vi "NIIE_LoadGraphics.vi"(4 "Templates User Event":refnum<user-event>, 6 "Glyphs User Event":refnum<user-event>, 8 "Error":errorcluster, 9 "Source":T1=enum."Icon Templates VI", 10 "Check Template?":bool, 11 "Graphic Root Folder":path) -> (0 "Error Out":errorcluster, 3 "Glyphs Out":T2[](array[typedef]), 5 "Match? Out":bool, 7 "Match Index Out":i32)   [LabVIEW 2021]
uses:
  MB CORE/TypeDefs/Cluster_Path&Icon.ctl
  vi.lib/LabVIEW Icon API/lv_icon/Controls/Pathes.ctl
  MB CORE/TypeDefs/Cluster_IconFilename.ctl
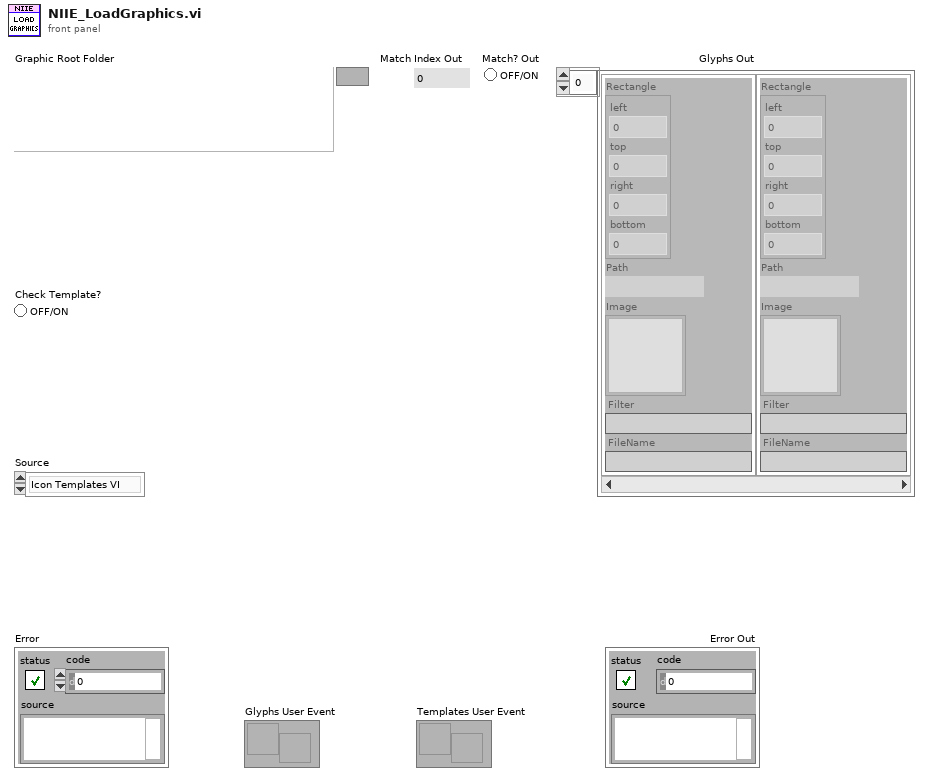
[diagram p1: front panel]
types:
  T1 = typedef "Pathes.ctl" = enum16{"Root Path", "Icon Templates", "Icon Templates VI", "Icon Templates Lib", "Glyphs"}
  T2 = typedef "Cluster_Path&Icon.ctl" = cluster{"Rectangle":cluster{"left":i16, "top":i16, "right":i16, "bottom":i16}, "Path":path, "Image":picture, "Filter":string, "FileName":string}
  T3 = typedef "Cluster_IconFilename.ctl" = cluster{"Name":string, "File Extension  ":string, "Filter":string, "Path":path}
  T4 = typedef "LabVIEW Icon Stored Information.ctl" = cluster{"Text Visible?":bool, "Text Opacity":u8, "Templ Visible?":bool, "Templ Opacity":u8, "Relative Path from 1 to 2":path, "Image":picture, "All User Layers":refnum<class "Layer.lvclass">[], "Body Text":T5}
  T5 = typedef "Cluster_BodyText.ctl" = cluster{"Line 1 text":string, "Line 2 text":string, "Line 3 text":string, "Line 4 text":string, "Line 1 color":u32, "Line 2 color":u32, "Line 3 color":u32, "Line 4 color":u32, "Body Text Spec":cluster{"Font":T6, "Alignment":T7, "Size":u8}, "Center text vertically":bool, "Capitalize Text":bool}
  T6 = typedef "Font.ctl" = string
  T7 = typedef "Alignment.ctl" = u16
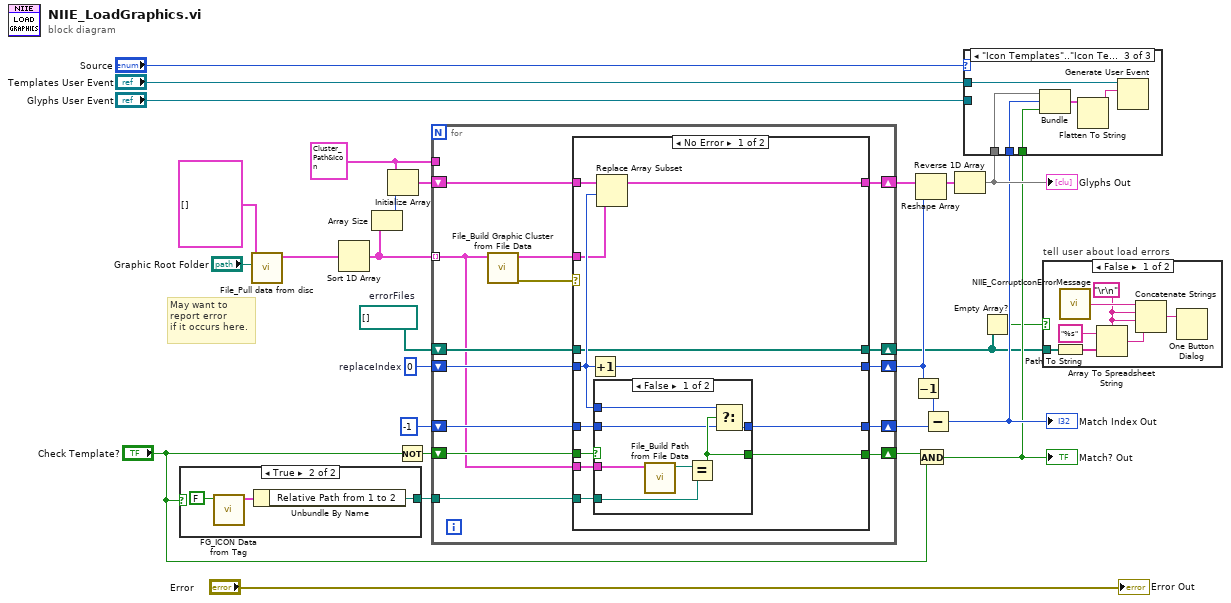
[diagram p0: block diagram]
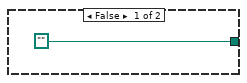
[diagram p2: hidden frame]
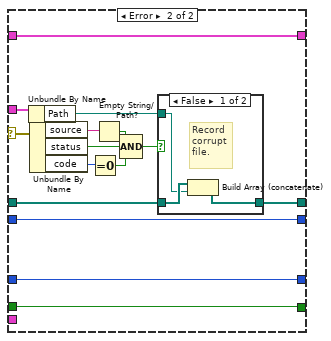
[diagram p4: hidden frame]
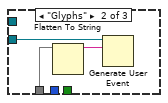
[diagram p8: hidden frame]
diagram:
  w6 = 0  # replaceIndex
  w7 = path[] []  # errorFiles
  w9 = T2 {"Rectangle"={"left"=0, "top"=0, "right"=0, "bottom"=0}, "Path"=path "", "Image"=bytes[0], "Filter"="", "FileName"=""} ("Path and Icon")
  # "May want to\nreport error\nif it occurs here."
  n1 = case shown="True" "Check Template?" {
    tunnel: [path "" w31] -> w12
    frame False {
    }
    frame True {
      n2 = call "FG_ICON Data from Tag.vi"("Init? (F)"=FALSE) -> ("Data Out"=w32:T4)  [unwired: 2 in, 8 out]
      n3 = Unbundle By Name(w32) -> ("Relative Path from 1 to 2"=w31:path)
    }
  }
  n4 = call "File_Pull data from disc.vi"("Graphic Root Folder"="Graphic Root Folder", "Data"=T3[] [] ("Data in")) -> ("Data Out"=w11:T3[])  [unwired: 1 in, 8 out]
  n5 = Sort 1D Array(array=w11) -> (sorted array=w27:T3[])
  n6 = Array Size(array=w27) -> (size(s)=w28:i32)
  n7 = Initialize Array(w9, w28) -> (w26:T2[])
  n8 = Not(x="Check Template?") -> (.not. x?=w24:bool)
  n9 = for {
    tunnel: w27 -> [w34] mode=indexing
    shift-right: [w35] -> w1
    shift-left: w7 -> [w36]
    shift-right: [w45] -> w25
    shift-left: w26 -> [w46]
    shift-right: [w42] -> w19
    shift-left: w24 -> [w44]
    tunnel: w12 -> [w43]
    shift-right: [w41] -> w22
    shift-left: -1 -> [w40]
    tunnel: w9 -> [_]
    shift-right: [w38] -> w3
    shift-left: w6 -> [w39]
    n10 = call "File_Build Graphic Cluster from File Data.vi"("File Data"=w34) -> ("Error Out"=w37:errorcluster, "Path And Icon Out"=w33:T2)  [unwired: 9 in]
    n11 = case shown="No Error" w37 {
      selector: w37 -> [_ w81]
      tunnel: w46 -> [w58 w82]
      tunnel: [w57 w82] -> w45
      tunnel: w44 -> [w56 w76]
      tunnel: w43 -> [w55 _]
      tunnel: [w54 w76] -> w42
      tunnel: [w53 w77] -> w41
      tunnel: w40 -> [w52 w77]
      tunnel: w39 -> [w51 w78]
      tunnel: [w50 w78] -> w38
      tunnel: w36 -> [w49 w74]
      tunnel: [w49 w70] -> w35
      tunnel: w34 -> [w47 _]
      tunnel: w33 -> [w48 w69]
      frame No Error {
        n12 = Increment(x=w51) -> (x+1=w50:i32)
        n13 = case shown="False" w56 {
          selector: w56 -> [_ w67]
          tunnel: w55 -> [w65 _]
          tunnel: [w63 w67] -> w54
          tunnel: [w64 w66] -> w53
          tunnel: w51 -> [w62 _]
          tunnel: w52 -> [w61 w66]
          tunnel: w47 -> [w59 _]
          frame False {
            n14 = call "File_Build Path from File Data.vi"("File Data"=w59) -> ("appended path"=w60:path)  [unwired: 10 in]
            n15 = Equal?(x=w60, y=w65) -> (x = y?=w63:bool)
            n16 = Select(t=w62, s=w63, f=w61) -> (s? t:f=w64:i32)
          }
          frame True {
          }
        }
        n17 = Replace Array Subset(array=w58, new element=w48, index=w51) -> (w57:T2[])
      }
      frame Error {
        n18 = Unbundle By Name(w69) -> ("Path"=w68:path)
        n19 = Unbundle By Name(w81) -> ("source"=w80:string, "status"=w72:bool, "code"=w79:i32)
        n20 = Equal To 0?(x=w79) -> (x = 0?=w73:bool)
        n21 = Empty String/Path?(string/path=w80) -> (empty?=w75:bool)
        n22 = Compound Arithmetic op=AND(w75, w72, w73) -> (w71:bool)
        n23 = case shown="False" w71 {
          tunnel: w74 -> [w85 w86]
          tunnel: [w83 w86] -> w70
          tunnel: w68 -> [w84 _]
          frame False {
            # "Record\ncorrupt\nfile."
            n24 = Build Array (concatenate)(w85, w84) -> (w83:path[])
          }
          frame True {
            # "Unsupported\nfile\nextension -\nignore it."
          }
        }
      }
    }
  }
  n25 = Decrement(x=w3) -> (x-1=w5:i32)
  n26 = Reshape Array(w25, w3) -> (w4:T2[])
  n27 = And(x=w19, y="Check Template?") -> (x .and. y?=w18:bool)
  "Match? Out" <- w18
  n28 = Subtract(x=w5, y=w22) -> (x-y=w20:i32)
  "Match Index Out" <- w20
  n29 = Reverse 1D Array(array=w4) -> (reversed array=w21:T2[])
  "Glyphs Out" <- w21
  n30 = case shown="\"Icon Templates\"..\"Icon Templates Lib\"" "Source" {
    tunnel: w21 -> [_ w88 w92]
    tunnel: w20 -> [_ _ w91]
    tunnel: w18 -> [_ _ w94]
    tunnel: "Glyphs User Event" -> [_ w87 _]
    tunnel: "Templates User Event" -> [_ _ w90]
    frame "Root Path", Default {
    }
    frame "Glyphs" {
      n31 = Flatten To String(anything=w88) -> (data string=w89:string)  [unwired: 1 in, 4 out]
      n32 = Generate User Event(user event=w87, event data cluster=w89) -> ()  [unwired: 2 in, 2 out]
    }
    frame "Icon Templates".."Icon Templates Lib" {
      n33 = Bundle(w92, w91, w94) -> (w93:cluster{T2[], i32, bool})  [unwired: 1 out]
      n34 = Flatten To String(anything=w93) -> (data string=w95:string)  [unwired: 1 in, 4 out]
      n35 = Generate User Event(user event=w90, event data cluster=w95) -> ()  [unwired: 2 in, 2 out]
    }
  }
  n36 = Empty Array?(array=w1) -> (empty?=w2:bool)
  n37 = case "tell user about load errors" shown="False" w2 {
    tunnel: w1 -> [w101 _]
    frame False {
      w99 = "\r\n"
      n38 = Path To String(path=w101) -> (string=w96:string[])
      n39 = call "NIIE_CorruptIconErrorMessage.vi"() -> ("corruptIconErrorMsg"=w102:string)  [unwired: 1 in]
      n40 = Array To Spreadsheet String(delimiter (Tab)=w99, array=w96, 3:"%s" ("format string")) -> (spreadsheet string=w98:string)
      n41 = Concatenate Strings(w102, w99, w99, w98) -> (w97:string)
      n42 = One Button Dialog(message=w97) -> ()  [unwired: 1 in, 1 out]
    }
    frame True {
    }
  }
  "Error Out" <- "Error"
